vi "Publish display files.vi"(11 "Method Name":string) -> (2 "Display images":string, 3 "Publish files":string)   [LabVIEW 2012]
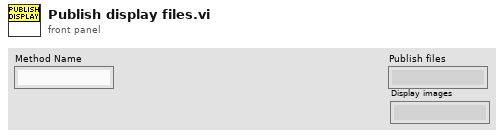
[diagram p1: front panel]
types:
  T1 = typedef "Method.ctl" = cluster{"Title":string, "About":string, "Input Parameters":cluster{"Description":string, "Name":string, "Min":string, "Max":string, "Default":string, "Units":string, "Increment":string, "Stock designs":string[]}[], "AutoCAD drawings":cluster{"File Name":string, "AC Variables":string[]}[], "Stock file names":string[], "Publish files":string[], "Display images":string[]}
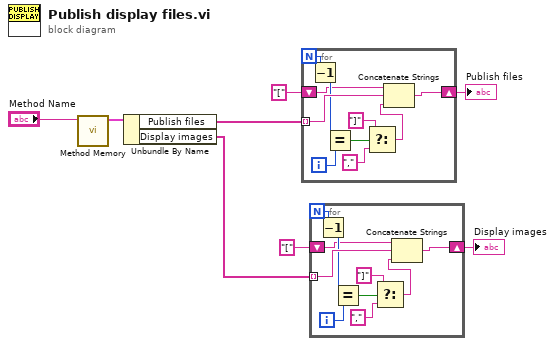
[diagram p0: block diagram]
diagram:
  n1 = call "Method Memory.vi"("Method Name"="Method Name") -> ("Method Out"=w8:T1)  [unwired: 8 in, 2 out]
  n2 = Unbundle By Name(w8) -> ("Publish files"=w7:string[], "Display images"=w3:string[])
  n3 = for {
    N -> [w16]
    tunnel: w7 -> [w18] mode=indexing
    shift-right: [w10] -> w2
    shift-left: "[" ("String") -> [w9]
    i -> [w17]
    n4 = Decrement(x=w16) -> (x-1=w15:i32)
    n5 = Equal?(x=w15, y=w17) -> (x = y?=w14:bool)
    n6 = Select(t="]" ("String"), s=w14, f="," ("String")) -> (s? t:f=w13:string)
    n7 = Concatenate Strings(w9, w18, w13) -> (w10:string)
  }
  "Publish files" <- w2
  n8 = for {
    N -> [w26]
    tunnel: w3 -> [w28] mode=indexing
    shift-right: [w20] -> w1
    shift-left: "[" ("String") -> [w19]
    i -> [w27]
    n9 = Decrement(x=w26) -> (x-1=w25:i32)
    n10 = Equal?(x=w25, y=w27) -> (x = y?=w24:bool)
    n11 = Select(t="]" ("String"), s=w24, f="," ("String")) -> (s? t:f=w23:string)
    n12 = Concatenate Strings(w19, w28, w23) -> (w20:string)
  }
  "Display images" <- w1
